vi "write error message.vi"(8 "error in":errorcluster) -> (3 "element":refnum<class "communicator message.lvclass">)   [LabVIEW 2015, in "communicator.lvclass"]
uses:
  communicator.lvclass
  message/communicator message.lvclass
  message/communicator message.lvclass/communicator message.ctl
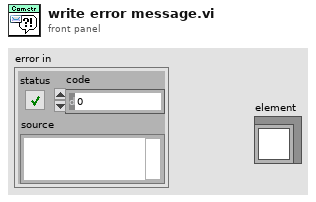
[diagram p1: front panel]
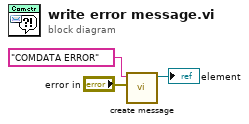
[diagram p0: block diagram]
diagram:
  n1 = call "create message.vi"("data"="error in", "ID"="COMDATA ERROR") -> ("message"=→"element":refnum<class "communicator message.lvclass">)  [unwired: 9 in]
